vi "Open Loop Gain Tool .vi"() -> ()   [LabVIEW 2018]
uses:
  <vilib>/DAQmx/write.llb/DAQmx Write (Digital Bool 1Line 1Point).vi
  <vilib>/DAQmx/read.llb/DAQmx Read (Analog DBL 1Chan 1Samp).vi
  <vilib>/DAQmx/create/channels.llb/DAQmx Create Channel (AI-Voltage-Basic).vi
  <vilib>/DAQmx/miscellaneous.llb/DAQmx Fill In Error Info.vi
  <vilib>/DAQmx/create/channels.llb/DAQmx Create Channel (DO-Digital Output).vi
  <vilib>/addons/control/pid/pid.llb/PID Gain Schedule (DBL).vi
  <vilib>/addons/control/pid/autopid.llb/PID Online Autotuning (Step Open Loop).vi
  <vilib>/addons/control/pid/pid.llb/PID Advanced (DBL).vi
  <vilib>/addons/control/pid/NI_PID_pid.lvlib
  <vilib>/ptbypt/NI_PtbyPt.lvlib
  <vilib>/addons/control/pid/NI_PID_autopid.lvlib
panel:
  out "TTL":bool
  out "Scaled MV":dbl(slide) scale=0.0..2000.0
  in  "Target Pressure(in Torr)":dbl
  out "Pressure Readout  (in Torr)":dbl(slide) scale=0.0..1000.0
  out "Pressure (in torr)":dbl
  in  "Sampling Time dt (s)":dbl=0.05 min=0.001 step=0.01 format="%#.3p"
  in  "Stop":bool
  out "SP and PV":cluster{"initial PV":dbl, "SP1:":dbl}(graph)={"initial PV"=50.98160323470328, "SP1:"=50.98039215686275}
  out "PID Gains":T1={"proportional gain (Kc)"=6.925505792902687, "integral time (Ti, min)"=0.004930412653813362, "derivative time (Td, min)"=0.0} {"derivative time (Td, min)" format="%#.6g"; "integral time (Ti, min)" format="%#.6g"; "proportional gain (Kc)" format="%#.6g"}
  in  "Autotune":bool
  in  "Replace gains":bool
  out "MV":dbl(graph)
  out "tuned PID gains":T1={"proportional gain (Kc)"=1.9838195929127882, "integral time (Ti, min)"=0.01995856284686879, "derivative time (Td, min)"=0.0} {"derivative time (Td, min)" format="%#.6g"; "integral time (Ti, min)" format="%#.6g"; "proportional gain (Kc)" format="%#.6g"}
  in  "autotuning parameters":T2={"Type of Controller"=2, "relay cycles"=3, "amplitude"=1.0, "control specifications"=2, "PV noise level"=0.1} {"PV noise level" format="%.2f"; "control specifications" items=["fast", "normal", "slow"]; "amplitude" format="%.2f"; "Type of Controller" items=["P", "PI", "PID"]}
  in  "Reinitialize":bool
  in  "Automatic":bool=TRUE
  in  "alpha":dbl=nan format="%.2f"
  in  "PID gain schedule":T3(array[cluster])=[{"PID gains"={"Kc"=7.0, "Ti"=0.001, "Td"=0.0}, "max value"=0.0}] {"max value" format="%.2f"; "PID gains"."Td" format="%#.3g"; "PID gains"."Ti" format="%#.3g"; "PID gains"."Kc" format="%#.3g"}
  in  "Insert gains":bool
  out "Gain Scheduling":i32
  # "Gain Scheduling"
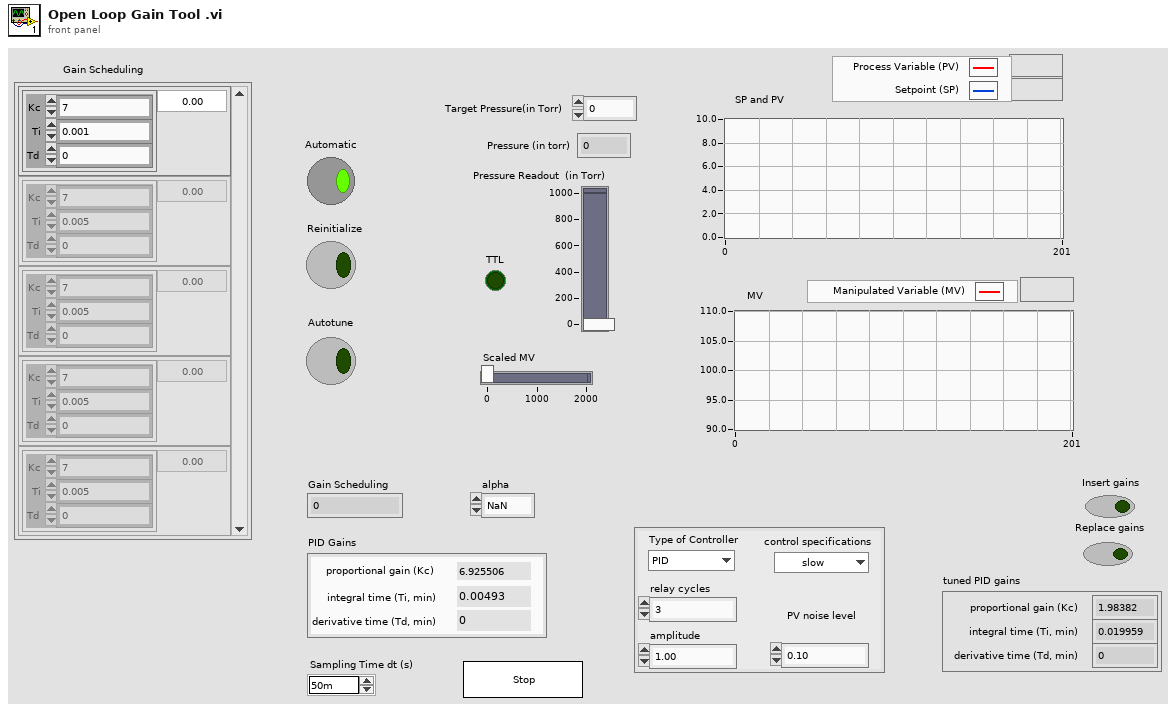
[diagram p1: front panel]
types:
  T1 = cluster{"proportional gain (Kc)":dbl, "integral time (Ti, min)":dbl, "derivative time (Td, min)":dbl}
  T2 = cluster{"Type of Controller":u16, "relay cycles":i32, "amplitude":dbl, "control specifications":u16, "PV noise level":dbl}
  T3 = cluster{"PID gains":cluster{"Kc":dbl, "Ti":dbl, "Td":dbl}, "max value":dbl}[]
  T4 = cluster{"tuned PID gains":cluster{"proportional gain (Kc)":dbl, "integral time (Ti, min)":dbl, "derivative time (Td, min)":dbl}, "Target Pressure(in Torr)":dbl}
  T5 = cluster{"PID gains":cluster{"Kc":dbl, "Ti":dbl, "Td":dbl}, "max value":dbl}
  T6 = cluster{"tuned PID gains":cluster{"proportional gain (Kc)":dbl, "integral time (Ti, min)":dbl, "derivative time (Td, min)":dbl}, "max value":dbl}
  T7 = cluster{"Pressure Readout  (in Torr)":dbl, "Target Pressure(in Torr)":dbl}
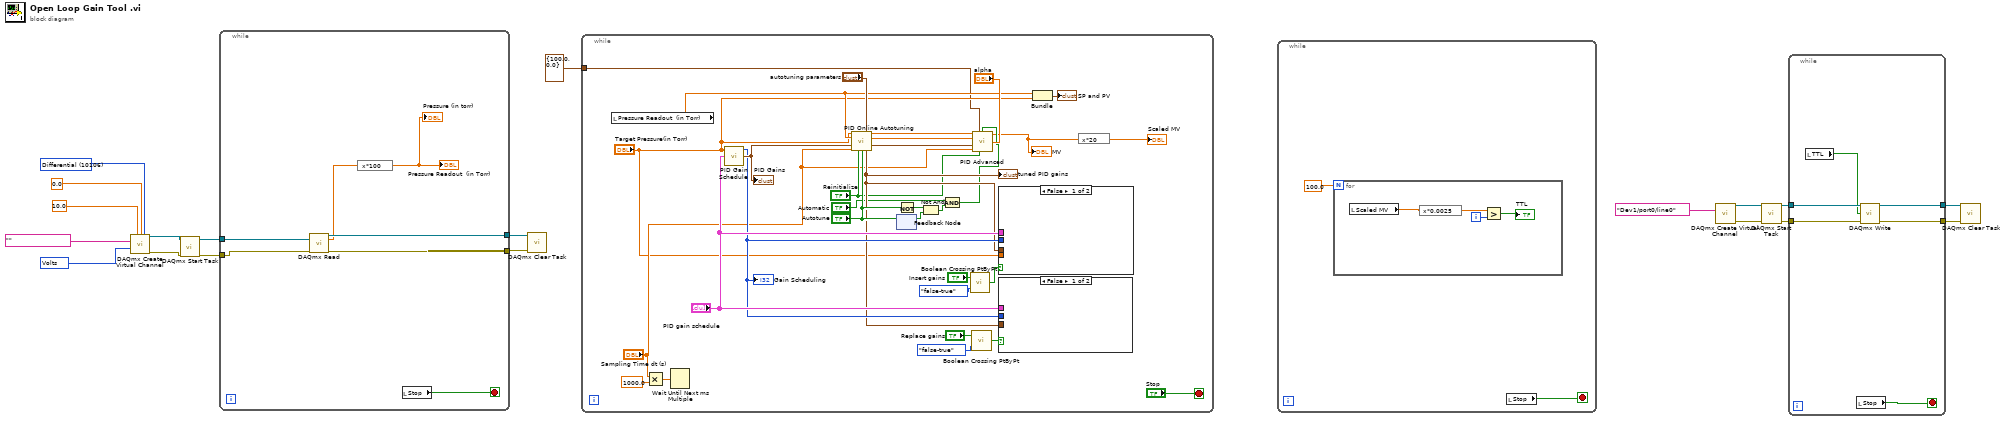
[diagram p0: block diagram]
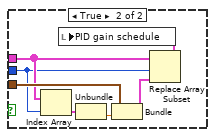
[diagram p2: hidden frame]
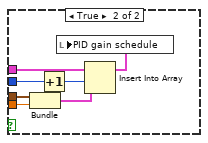
[diagram p3: hidden frame]
diagram:
  w9 = 10348 items=["Volts"=10348, "From Custom Scale"=10065] ("units")
  w11 = 10106 items=["Default"=-1, "RSE"=10083, "NRSE"=10078, "Differential"=10106, "Pseudodifferential"=12529] ("input terminal configuration")
  n1 = call-poly <vilib>:"DAQmx Create Virtual Channel.vi"("maximum value"=10.0, "minimum value"=0.0, "input terminal configuration"=w11, "physical channels"=tag "", "units"=w9) -> ("task out"=w19:refnum<k21>, "error out"=w18:errorcluster)  [unwired: 9 in]
  n2 = call <vilib>:"DAQmx Start Task.vi"("task/channels in"=w19, "error in"=w18) -> ("task out"=w17:refnum<k21>, "error out"=w15:errorcluster)  [unwired: 12 in]
  n3 = while {
    tunnel: w17 -> [w26]
    tunnel: [w25] -> w16
    tunnel: w15 -> [w24]
    tunnel: [w23] -> w14
    stop <- w20 stop-if-true
    n4 = call-poly <vilib>:"DAQmx Read.vi"("task/channels in"=w26, "error in"=w24) -> ("task out"=w25:refnum<k21>, "data"=w22:dbl, "error out"=w23:errorcluster)  [unwired: 11 in]
    n5 = expression code="x*100"(w22) -> (→"Pressure Readout  (in Torr)" →"Pressure (in torr)":dbl)
    n6 = local read "Stop"() -> (w20:bool)
  }
  n7 = call <vilib>:"DAQmx Clear Task.vi"("task in"=w16, "error in"=w14) -> ()  [unwired: 13 in, 1 out]
  n8 = while {
    tunnel: cluster{"output high":dbl, "output low":dbl} {"output high"=100.0, "output low"=0.0} ("output range") -> [w27]
    stop <- "Stop" stop-if-true
    n9 = local read "Pressure Readout  (in Torr)"() -> (w35:dbl)
    n10 = Multiply(x="Sampling Time dt (s)", y=1000.0) -> (x*y=w33:dbl)
    n11 = Wait Until Next ms Multiple(millisecond multiple=w33) -> ()  [unwired: 1 out]
    n12 = call-poly <vilib>:"PID Gain Schedule.vi"("PID gain schedule"="PID gain schedule", "gain scheduling value"="Target Pressure(in Torr)") -> ("PID gains out"=w47:T1, "index out"=w42:i32)  [unwired: 2 in]
    "PID Gains" <- w47
    "Gain Scheduling" <- w42
    n13 = call-poly <vilib>:"PID Online Autotuning.vi"("setpoint"="Target Pressure(in Torr)", "autotuning parameters"="autotuning parameters", "process variable"=w35, "PID gains in"=w47, "dt (s)"="Sampling Time dt (s)", "reinitialize? (F)"="Reinitialize", "autotune? (F)"="Autotune") -> ("setpoint out"=w57:dbl, "process variable out"=w56:dbl, "PID gains out"=w54:T1, "tuned PID gains"=w41:T1)  [unwired: 4 in, 1 out]
    "tuned PID gains" <- w41
    n14 = feedback #1() -> (w53:bool)  [unwired: 1 in]
    n15 = feedback-in #1("Autotune") -> ()
    n16 = Not(x="Autotune") -> (.not. x?=w50:bool)
    n17 = Not And(1:w53, 2:w50) -> (0:w51:bool)
    n18 = And(x="Automatic", y=w51) -> (x .and. y?=w38:bool)
    n19 = call <vilib>:"Boolean Crossing PtByPt.vi"("direction"=enum16{"either", "false-true", "true-false"}."false-true", "input"="Insert gains") -> ("crossing"=w48:bool)  [unwired: 1 in]
    n20 = call <vilib>:"Boolean Crossing PtByPt.vi"("direction"=enum16{"either", "false-true", "true-false"}."false-true", "input"="Replace gains") -> ("crossing"=w44:bool)  [unwired: 1 in]
    n21 = call-poly <vilib>:"PID Advanced.vi"("setpoint"=w57, "output range"=w27, "auto? (T)"=w38, "process variable"=w56, "alpha"="alpha", "PID gains"=w54, "dt (s)"="Sampling Time dt (s)", "reinitialize? (F)"="Reinitialize") -> ("output"=w29:dbl)  [unwired: 6 in, 1 out]
    "MV" <- w29
    n22 = case shown="False" w48 {
      tunnel: w41 -> [_ w72]
      tunnel: "Target Pressure(in Torr)" -> [_ w71]
      tunnel: "PID gain schedule" -> [_ w69]
      tunnel: w42 -> [_ w67]
      frame False {
      }
      frame True {
        n23 = Bundle("tuned PID gains"=w72, "Target Pressure(in Torr)"=w71) -> (w70:T4)  [unwired: 1 in]
        n24 = Increment(x=w67) -> (x+1=w66:i32)
        n25 = Insert Into Array(array=w69, index=w66, new element=w70) -> (w68:T3)
        n26 = local write "PID gain schedule"(w68) -> ()
      }
    }
    n27 = case shown="False" w44 {
      tunnel: w41 -> [_ w65]
      tunnel: "PID gain schedule" -> [_ w62]
      tunnel: w42 -> [_ w61]
      frame False {
      }
      frame True {
        n28 = Index Array(array=w62, index=w61) -> (element=w60:T5)
        n29 = Unbundle(w60) -> ("max value"=w59:dbl)  [unwired: 1 out]
        n30 = Bundle("tuned PID gains"=w65, "max value"=w59) -> (w63:T6)  [unwired: 1 in]
        n31 = Replace Array Subset(array=w62, new element=w63, index=w61) -> (w64:T3)
        n32 = local write "PID gain schedule"(w64) -> ()
      }
    }
    n33 = Bundle("Pressure Readout  (in Torr)"=w35, "Target Pressure(in Torr)"="Target Pressure(in Torr)") -> (→"SP and PV":T7)  [unwired: 1 in]
    n34 = expression code="x*20"(w29) -> (→"Scaled MV":dbl)
  }
  n35 = while {
    stop <- w73 stop-if-true
    n36 = for {
      N: 100.0 -> [_]
      i -> [w78]
      n37 = local read "Scaled MV"() -> (w75:dbl)
      n38 = expression code="x*0.0025"(w75) -> (w77:dbl)
      n39 = Greater?(x=w77, y=w78) -> (0:→"TTL":bool)
    }
    n40 = local read "Stop"() -> (w73:bool)
  }
  n41 = call-poly <vilib>:"DAQmx Create Virtual Channel.vi"("lines"=tag "Dev1/port0/line0") -> ("task out"=w5:refnum<k21>, "error out"=w4:errorcluster)  [unwired: 13 in]
  n42 = call <vilib>:"DAQmx Start Task.vi"("task/channels in"=w5, "error in"=w4) -> ("task out"=w3:refnum<k21>, "error out"=w2:errorcluster)  [unwired: 12 in]
  n43 = while {
    tunnel: [w84] -> w8
    tunnel: [w83] -> w7
    tunnel: w3 -> [w82]
    tunnel: w2 -> [w81]
    stop <- w79 stop-if-true
    n44 = local read "TTL"() -> (w80:bool)
    n45 = local read "Stop"() -> (w79:bool)
    n46 = call-poly <vilib>:"DAQmx Write.vi"("task/channels in"=w82, "data"=w80, "error in"=w81) -> ("task out"=w84:refnum<k21>, "error out"=w83:errorcluster)  [unwired: 10 in, 1 out]
  }
  n47 = call <vilib>:"DAQmx Clear Task.vi"("task in"=w8, "error in"=w7) -> ()  [unwired: 13 in, 1 out]
